vi "Seg1_Charging_Limit_current_checking.vi"(5 "File_name":string, 6 "Numeric in":i32, 7 "Stop Current(A) after Full":dbl, 8 "error in (no error)":errorcluster, 9 "Log?":bool, 10 "Numeric 3":i32, 11 "VISA Refnum in":refnum<visa-resource-name>) -> (0 "error out":errorcluster, 1 "Peak to Peak 2 (Curr)":dbl, 2 "Boolean":bool, 3 "VISA Refnum out":refnum<visa-resource-name>, 4 "Peak to Peak (vol)":dbl)   [LabVIEW 2015]
uses:
  <vilib>/Utility/file.llb/Write Delimited Spreadsheet (string).vi
  <instrlib>/Agilent N6700 Series/Agilent N6700 Series.lvlib
panel:
  in  "Index":i32
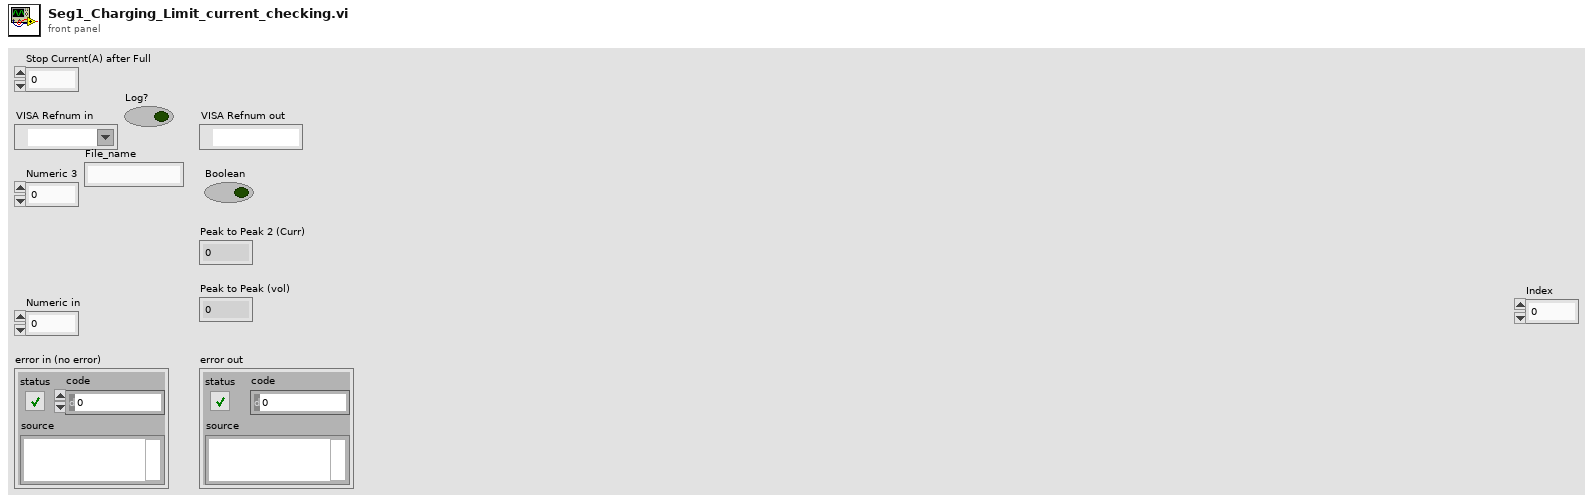
[diagram p1: front panel]
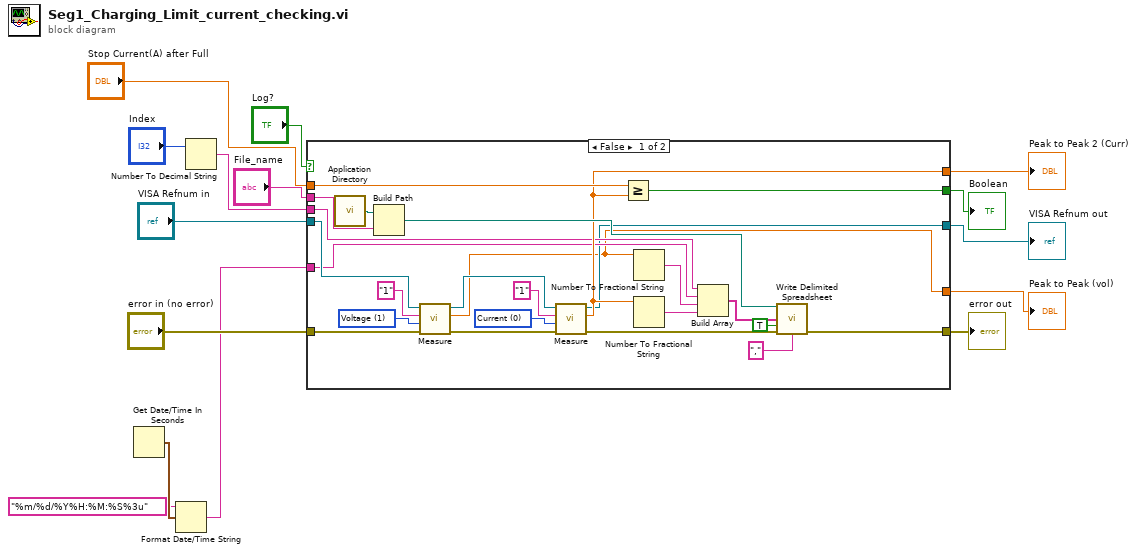
[diagram p0: block diagram]
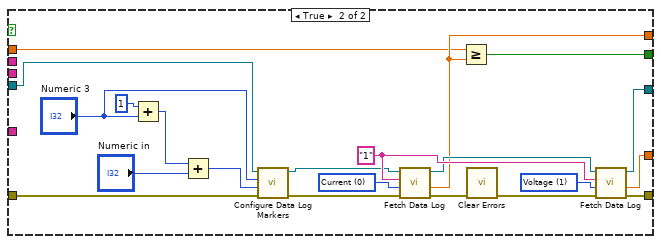
[diagram p2: hidden frame]
diagram:
  n1 = Get Date/Time In Seconds() -> (seconds since 1Jan1904=w3:timestamp)
  n2 = Format Date/Time String(time format string (%c)="%m/%d/%Y%H:%M:%S%3u", seconds (now)=w3) -> (date/time string=w1:string)  [unwired: 1 in]
  n3 = Number To Decimal String(number="Index") -> (decimal integer string=w4:string)  [unwired: 1 in]
  n4 = case shown="False" "Log?" {
    tunnel: [w17 w61] -> w15
    tunnel: [w24 w59] -> w14
    tunnel: [w18 w58] -> w13
    tunnel: [w21 w54] -> w12
    tunnel: "Stop Current(A) after Full" -> [w23 w53]
    tunnel: [w22 w49] -> w10
    tunnel: "error in (no error)" -> [w25 w47]
    tunnel: "VISA Refnum in" -> [w26 w45]
    tunnel: "File_name" -> [w27 _]
    tunnel: w4 -> [w20 _]
    tunnel: w1 -> [w19 _]
    frame False {
      w32 = 0 items=["Current", "Voltage", "Power"] ("Measurement Type (1: Voltage)")
      w33 = 1 items=["Current", "Voltage", "Power"] ("Measurement Type (1: Voltage)")
      n5 = call <vilib>:"Application Directory.vi"() -> ("Application Directory"=w35:path)
      n6 = Build Path(base path=w35, name or relative path=w27) -> (appended path=w34:path)
      n7 = call <instrlib>:"Measure.vi"("error in (no error)"=w25, "Measurement Type (1: Voltage)"=w33, "Channel Name (1)"="1", "VISA resource name"=w26) -> ("error out"=w28:errorcluster, "Measurement"=w17:dbl, "VISA resource name out"=w29:refnum<visa-resource-name>)  [unwired: 5 in]
      n8 = call <instrlib>:"Measure.vi"("error in (no error)"=w28, "Measurement Type (1: Voltage)"=w32, "Channel Name (1)"="1", "VISA resource name"=w29) -> ("error out"=w38:errorcluster, "Measurement"=w21:dbl, "VISA resource name out"=w18:refnum<visa-resource-name>)  [unwired: 5 in]
      n9 = Greater Or Equal?(x=w23, y=w21) -> (x >= y?=w22:bool)
      n10 = Number To Fractional String(number=w17) -> (F-format string=w39:string)  [unwired: 3 in]
      n11 = Number To Fractional String(number=w21) -> (F-format string=w40:string)  [unwired: 3 in]
      n12 = Build Array(w20, w19, w39, w40) -> (w37:string[])
      n13 = call-poly <vilib>:"Write Delimited Spreadsheet.vi"("file path (dialog if empty)"=w34, "1D data"=w37, "append to file? (F)"=TRUE, "error in (no error)"=w38, "delimiter (\\t)"="," ("delimiter (\\t)")) -> ("error out"=w24:errorcluster)  [unwired: 9 in, 1 out]
    }
    frame True {
      w57 = 1 items=["Voltage"=1, "Current"=0] ("Data Log Type (1: Voltage)")
      w43 = 0 items=["Voltage"=1, "Current"=0] ("Data Log Type (1: Voltage)")
      w56 = "1" ("Channel Name (1)")
      n14 = Add(x=1, y="Numeric 3") -> (x+y=w51:i32)
      n15 = Add(x=w51, y="Numeric in") -> (x+y=w52:i32)
      n16 = call <instrlib>:"Configure Data Log Markers.vi"("error in (no error)"=w47, "Data Log Marker 2 (27.5 s)"=w52, "Data Log Marker 1 (7.5 s)"="Numeric 3", "VISA resource name"=w45) -> ("error out"=w46:errorcluster, "VISA resource name out"=w44:refnum<visa-resource-name>)  [unwired: 6 in]
      n17 = call <instrlib>:"Fetch Data Log.vi"("error in (no error)"=w46, "Data Log Type (1: Voltage)"=w43, "Channel Name (1)"=w56, "VISA resource name"=w44) -> ("error out"=w48:errorcluster, "Peak to Peak"=w54:dbl, "VISA resource name out"=w55:refnum<visa-resource-name>)  [unwired: 5 in]
      n18 = Greater Or Equal?(x=w53, y=w54) -> (x >= y?=w49:bool)
      n19 = call <vilib>:"Clear Errors.vi"("error in (no error)"=w48) -> ("error out"=w60:errorcluster)  [unwired: 5 in, 1 out]
      n20 = call <instrlib>:"Fetch Data Log.vi"("error in (no error)"=w60, "Data Log Type (1: Voltage)"=w57, "Channel Name (1)"=w56, "VISA resource name"=w55) -> ("error out"=w59:errorcluster, "Peak to Peak"=w61:dbl, "VISA resource name out"=w58:refnum<visa-resource-name>)  [unwired: 5 in]
    }
  }
  "Peak to Peak (vol)" <- w15
  "error out" <- w14
  "VISA Refnum out" <- w13
  "Peak to Peak 2 (Curr)" <- w12
  "Boolean" <- w10
